vi "P3.vi"() -> ()   [LabVIEW 2021]
uses:
  <vilib>/LabVIEW Interface for Arduino/Type Defs/Digital Pin.ctl
  <vilib>/LabVIEW Interface for Arduino/Type Defs/Board Type.ctl
  <vilib>/LabVIEW Interface for Arduino/Type Defs/Connection Type.ctl
  <vilib>/LabVIEW Interface for Arduino/Type Defs/Pin Mode.ctl
  <vilib>/LabVIEW Interface for Arduino/LabVIEW Interface for Arduino.lvlib
panel:
  in  "CERRAR PUERTO":bool
  out "ARRAY DATO LEIDO":bool[](array[boolean])
  in  "PIN DIGITAL":T1
  # "Practica 3: Leer una entrada digital"
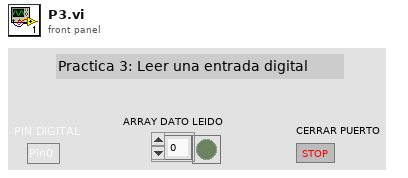
[diagram p1: front panel]
types:
  T1 = typedef "LabVIEW Interface for Arduino.lvlib/Digital Pin.ctl" = enum8{"Pin0", "Pin1", "Pin2", "Pin3", "Pin4", "Pin5", "Pin6", "Pin7", "Pin8", "Pin9", "Pin10", "Pin11", "Pin12", "Pin13"}
  T2 = typedef "LabVIEW Interface for Arduino.lvlib/Connection Type.ctl" = enum8{"USB / Serial", "XBEE", "BlueSmirf (Bluetooth)"}
  T3 = typedef "LabVIEW Interface for Arduino.lvlib/Board Type.ctl" = enum16{"Uno", "Dimuelanove w/Atmega 328", "Mega 2560"}
  T4 = typedef "LabVIEW Interface for Arduino.lvlib/Arduino Resource.ctl" = cluster{"VISA resource":refnum<visa-resource-name>, "Board Type":T3, "Connection Type":enum8{"USB / Serial"}, "Bytes Per Packet (15)":u8}
  T5 = typedef "LabVIEW Interface for Arduino.lvlib/Pin Mode.ctl" = enum8{"Input", "Output"}
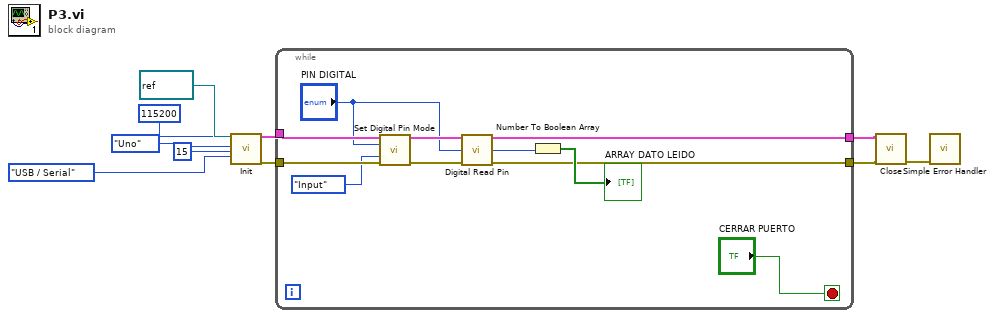
[diagram p0: block diagram]
diagram:
  n1 = call <vilib>:"Init.vi"("VISA resource"=refnum<visa-resource-name> "COM11", "Baud Rate (115200)"=u32 115200, "Board Type (Uno)"=Board_Type."Uno", "Bytes Per Packet (15)"=u32 15, "Connection Type (USB/Serial)"=Connection_Type."USB / Serial") -> ("Arduino Resource"=w5:T4, "error out"=w4:errorcluster)  [unwired: 13 in]
  n2 = while {
    tunnel: w5 -> [w20]
    tunnel: w4 -> [w19]
    tunnel: [w12] -> w3
    tunnel: [w11] -> w2
    stop <- "CERRAR PUERTO" stop-if-true
    n3 = call <vilib>:"Set Digital Pin Mode.vi"("Arduino Resource"=w20, "Digital I/O Pin"="PIN DIGITAL", "Pin Mode (Input)"=Pin_Mode."Input", "error in"=w19) -> ("Arduino Resource"=w17:T4, "error out"=w16:errorcluster)  [unwired: 10 in]
    n4 = call <vilib>:"Digital Read Pin.vi"("Arduino Resource"=w17, "Digital I/O Pin (0)"="PIN DIGITAL", "error in"=w16) -> ("Arduino Resource"=w12:T4, "Value"=w14:u8, "error out"=w11:errorcluster)  [unwired: 10 in]
    n5 = Number To Boolean Array(number=w14) -> (Boolean array=→"ARRAY DATO LEIDO":bool[])
  }
  n6 = call <vilib>:"Close.vi"("Arduino Resource"=w3, "error in"=w2) -> ("error out"=w1:errorcluster)  [unwired: 13 in]
  n7 = call <vilib>:"Simple Error Handler.vi"("error in (no error)"=w1) -> ()  [unwired: 4 in, 5 out]
